vi "OpenPrefDialog.vi"(8 "error in (no error)":errorcluster, 11 "INI File Path":path) -> (0 "error out":errorcluster)   [LabVIEW 2018, in "Test.lvclass"]
uses:
  Test.lvclass
  AcPwr/AcPwrPlugins/AcPwrBaseClass/AcPwrBase.lvclass
  Sensor/SensorPlugins/SensorBaseClass/SensorBase.lvclass
  Sync/SyncPlugins/SyncPluginBase/SyncPluginBase.lvclass
  FGen/FgenPlugins/FgenPluginBaseClass/FgenPluginsBase.lvclass
  Digitizer/DigitizerPlugins/DigitizerBaseClass/DigitizerBase.lvclass
  Analysis/AnalysisPlugins/AnalysisPluginBaseClass/AnalysisPluginsBase.lvclass
  Scope/ScopePlugins/ScopePluginBaseClass/ScopePluginsBase.lvclass
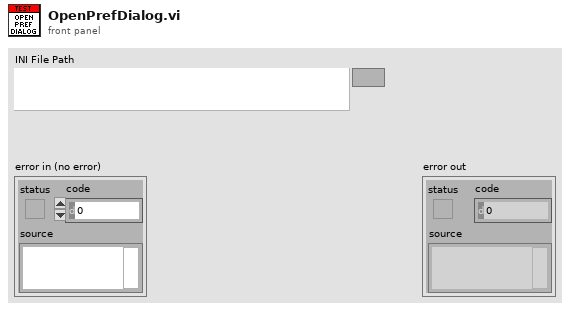
[diagram p1: front panel]
types:
  T1 = typedef "INIInfo.ctl" = cluster{"Module Name":string, "INI File Name":string, "Class Name":string, "INI File Name Without Extension":string, "Module.Class.INI File Name":string, "Visualization VI Path":path, "Instrument Class Path":path}
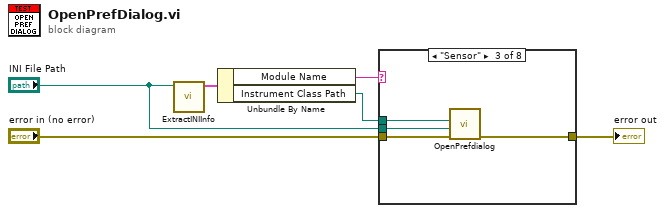
[diagram p0: block diagram]
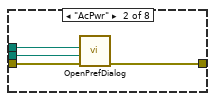
[diagram p3: hidden frame]
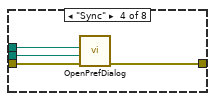
[diagram p4: hidden frame]
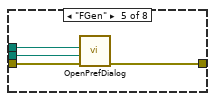
[diagram p5: hidden frame]
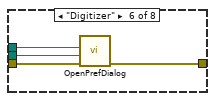
[diagram p6: hidden frame]
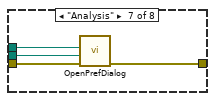
[diagram p7: hidden frame]
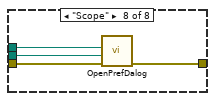
[diagram p8: hidden frame]
diagram:
  n1 = call "ExtractINIInfo.vi"("INI File Path"="INI File Path") -> ("INI Info"=w5:T1)  [unwired: 8 in, 2 out]
  n2 = Unbundle By Name(w5) -> ("Module Name"=w2:string, "Instrument Class Path"=w1:path)
  n3 = case shown="\"Sensor\"" w2 {
    tunnel: "INI File Path" -> [_ w10 w14 w18 w22 w26 w30 w31]
    tunnel: w1 -> [_ w9 w13 w17 w21 w25 w29 w32]
    tunnel: "error in (no error)" -> [_ w8 w12 w16 w20 w24 w28 w34]
    tunnel: [_ w7 w11 w15 w19 w23 w27 w33] -> w3
    frame "False", Default {
    }
    frame "AcPwr" {
      n4 = call "OpenPrefDialog.vi"("error in (no error)"=w8, "PluginIniFilePath"=w10, "Class Path"=w9) -> ("error out"=w7:errorcluster)  [unwired: 8 in]
    }
    frame "Sensor" {
      n5 = call "OpenPrefdialog.vi"("error in (no error)"=w12, "PluginIniFilePath"=w14, "Class Path"=w13) -> ("error out"=w11:errorcluster)  [unwired: 8 in]
    }
    frame "Sync" {
      n6 = call "OpenPrefDialog.vi"("error in (no error)"=w16, "PluginIniFilePath"=w18, "Class Path"=w17) -> ("error out"=w15:errorcluster)  [unwired: 8 in]
    }
    frame "FGen" {
      n7 = call "OpenPrefDialog.vi"("error in (no error)"=w20, "PluginIniFilePath"=w22, "Class Path"=w21) -> ("error out"=w19:errorcluster)  [unwired: 8 in]
    }
    frame "Digitizer" {
      n8 = call "OpenPrefDialog.vi"("error in (no error)"=w24, "PluginIniFilePath"=w26, "Class Path"=w25) -> ("error out"=w23:errorcluster)  [unwired: 8 in]
    }
    frame "Analysis" {
      n9 = call "OpenPrefDialog.vi"("error in (no error)"=w28, "PluginIniFilePath"=w30, "Class Path"=w29) -> ("error out"=w27:errorcluster)  [unwired: 8 in]
    }
    frame "Scope" {
      n10 = call "OpenPrefDalog.vi"("error in (no error)"=w34, "PluginIniFilePath"=w31, "Class Path"=w32) -> ("error out"=w33:errorcluster)  [unwired: 8 in]
    }
  }
  "error out" <- w3
